vi "Get Device Parameters.vi"(8 "error in":errorcluster, 11 "Ballard MIL-STD 1553 custom device in":T3=18446744073709551615 format="%.0x") -> (0 "error out":errorcluster, 2 "device parameters":T1, 3 "Ballard MIL-STD 1553 custom device out":T3 format="%.0x")   [LabVIEW 2020, in "AIM MIL-STD-1553 Scripting.lvlib"]
doc: "Returns Ballard hardware <b>device parameters</b> such as <b>PXI slot number</b> and <b>core number</b> as configured in the system definition. This VI does not perform device discovery."
uses:
  AIM MIL-STD-1553 Scripting.lvlib
  <vilib>/NI VeriStand/Custom Device API/Custom Device Item Ref.ctl
  Shared/Device Parameters.ctl
  Shared/Initialization Method.ctl
  Constants.vi
  <vilib>/NI VeriStand/Custom Device API/Get Item Property (U16).vi
  <vilib>/NI VeriStand/Custom Device API/Get Item Property (I32).vi
  <vilib>/NI VeriStand/Custom Device API/Custom Device API.lvlib
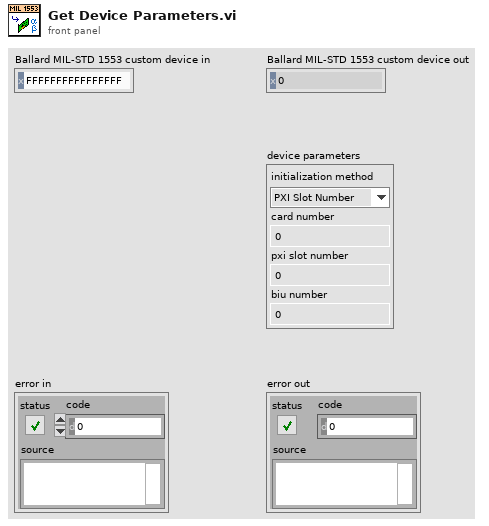
[diagram p1: front panel]
types:
  T1 = typedef "Device Parameters.ctl" = cluster{"initialization method":T2, "card number":i32, "pxi slot number":i32, "biu number":i32}
  T2 = typedef "Initialization Method.ctl" = enum16{"PXI Slot Number", "Card Number"}
  T3 = typedef "Custom Device API.lvlib/Custom Device Item Ref.ctl" = u64
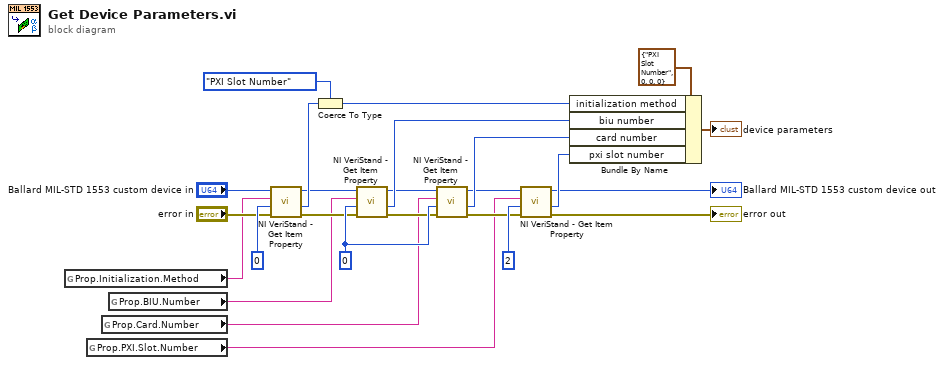
[diagram p0: block diagram]
diagram:
  w24 = 0 ("Default Value")
  n1 = global read "Constants.vi" "Prop.Initialization.Method"() -> (w7:string)
  n2 = global read "Constants.vi" "Prop.PXI.Slot.Number"() -> (w4:string)
  n3 = global read "Constants.vi" "Prop.Card.Number"() -> (w5:string)
  n4 = global read "Constants.vi" "Prop.BIU.Number"() -> (w6:string)
  n5 = call-poly <vilib>:"NI VeriStand - Get Item Property.vi"("error in (no error)"="error in", "Default Value"=u16 0, "Property Name"=w7, "Item Ref in"="Ballard MIL-STD 1553 custom device in") -> ("error out"=w12:errorcluster, "Value"=w19:u16, "Item Ref out"=w11:T3)  [unwired: 4 in, 1 out]
  n6 = Coerce To Type(0:w19, 1:Initialization_Method."PXI Slot Number" ("initialization method")) -> (2:w10:T2)
  n7 = call-poly <vilib>:"NI VeriStand - Get Item Property.vi"("error in (no error)"=w12, "Default Value"=w24, "Property Name"=w6, "Item Ref in"=w11) -> ("error out"=w17:errorcluster, "Value"=w22:i32, "Item Ref out"=w18:T3)  [unwired: 4 in, 1 out]
  n8 = call-poly <vilib>:"NI VeriStand - Get Item Property.vi"("error in (no error)"=w17, "Default Value"=w24, "Property Name"=w5, "Item Ref in"=w18) -> ("error out"=w15:errorcluster, "Value"=w21:i32, "Item Ref out"=w16:T3)  [unwired: 4 in, 1 out]
  n9 = call-poly <vilib>:"NI VeriStand - Get Item Property.vi"("error in (no error)"=w15, "Default Value"=2, "Property Name"=w4, "Item Ref in"=w16) -> ("error out"=→"error out":errorcluster, "Value"=w20:i32, "Item Ref out"=→"Ballard MIL-STD 1553 custom device out":T3)  [unwired: 4 in, 1 out]
  n10 = Bundle By Name(cluster=T1 {"initialization method"=enum."PXI Slot Number", "card number"=0, "pxi slot number"=0, "biu number"=0} ("device parameters"), "initialization method"=w10, "biu number"=w22, "card number"=w21, "pxi slot number"=w20) -> (→"device parameters":T1)
